vi "Delete CR in String.vi"(4 "Input String":string) -> (1 "String without CR":string)   [LabVIEW 2013]
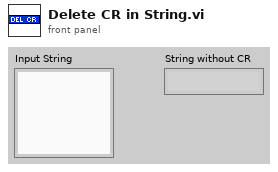
[diagram p1: front panel]
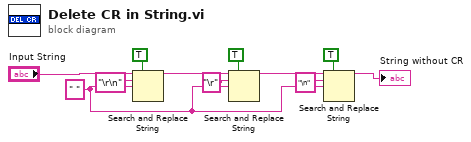
[diagram p0: block diagram]
diagram:
  w2 = " "
  n1 = Search and Replace String(replace all?=TRUE ("replace all? (F)"), input string="Input String", search string="\r\n", replace string=w2) -> (result string=w4:string)  [unwired: 1 in, 6 out]
  n2 = Search and Replace String(replace all?=TRUE ("replace all? (F)"), input string=w4, search string="\r", replace string=w2) -> (result string=w7:string)  [unwired: 1 in, 6 out]
  n3 = Search and Replace String(replace all?=TRUE ("replace all? (F)"), input string=w7, search string="\n", replace string=w2) -> (result string=→"String without CR":string)  [unwired: 1 in, 6 out]
